vi "cal_sub_numeric_string_pos.vi"(7 "Last Control  Position":cluster{"Left":i32, "Top":i32}, 9 "Last Function  Position":cluster{"Left":i32, "Top":i32}, 11 "error in":errorcluster) -> (8 "Ccontrol BD Position":cluster{"1st sub node x position":i32, i32}, 15 "error out":errorcluster)   [LabVIEW 2018]
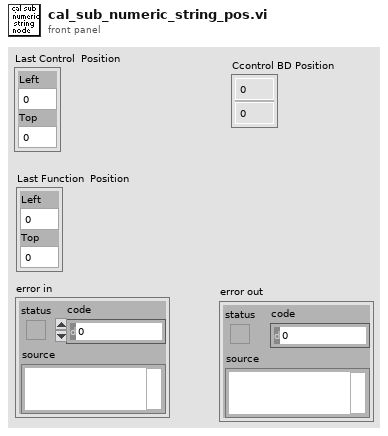
[diagram p1: front panel]
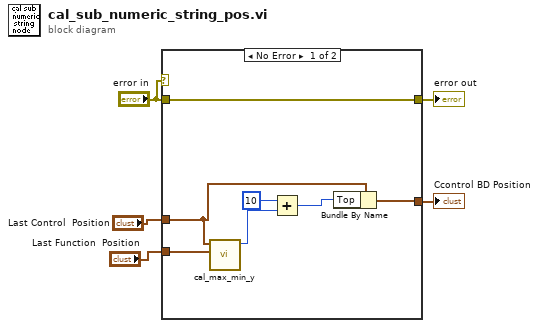
[diagram p0: block diagram]
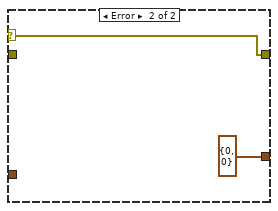
[diagram p2: hidden frame]
diagram:
  n1 = case shown="No Error" "error in" {
    selector: "error in" -> [_ w14]
    tunnel: [w6 w14] -> w5
    tunnel: "error in" -> [w6 _]
    tunnel: [w7 cluster{"1st sub node x position":i32, i32} {"1st sub node x position"=0, 0}] -> w4
    tunnel: "Last Control  Position" -> [w9 _]
    tunnel: "Last Function  Position" -> [w11 _]
    frame No Error {
      n2 = call "cal_max_min_y.vi"("Position 2"=w11, "Position 1"=w9) -> ("max y"=w10:i32)  [unwired: 9 out]
      n3 = Add(x=10, y=w10) -> (x+y=w12:i32)
      n4 = Bundle By Name(cluster=w9, "Top"=w12) -> (w7:cluster{"Left":i32, "Top":i32})
    }
    frame Error {
    }
  }
  "error out" <- w5
  "Ccontrol BD Position" <- w4
